vi "Wait if Occupied.vi"(9 "Desired Direction":T1, 10 "Desired Action":T2, 11 "Square":refnum<class "Square.lvclass">) -> (2 "Resulting Action":T2)   [LabVIEW 2020, in "SquareBattle.lvlib" / "Square.lvclass"]
uses:
  Square.lvclass
  Square.lvclass/Square.ctl
  Action.ctl
  SquareBattle.lvlib
  Direction.ctl
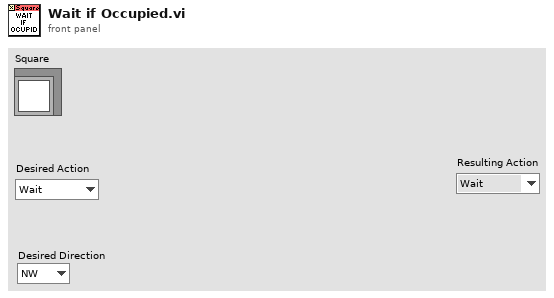
[diagram p1: front panel]
types:
  T1 = typedef "SquareBattle.lvlib/Direction.ctl" = enum16{"NW", "N", "NE", "E", "SE", "S", "SW", "W"}
  T2 = typedef "SquareBattle.lvlib/Action.ctl" = enum16{"Wait", "Move", "Attack", "Replicate"}
  T3 = typedef "SquareBattle.lvlib/Location Status.ctl" = cluster{"Empty":bool, "Friend":bool, "Enemy":bool}
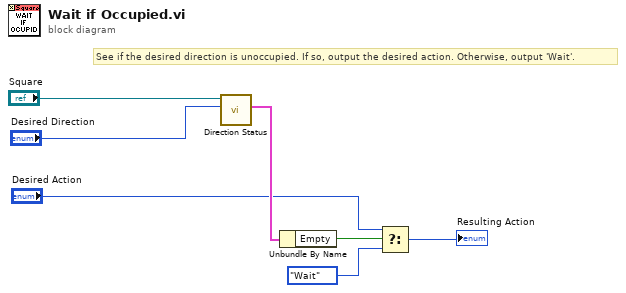
[diagram p0: block diagram]
diagram:
  # "See if the desired direction is unoccupied. If so, output the desired action. Otherwise, output 'Wait'."
  n1 = call "Direction Status.vi"("Direction"="Desired Direction", "Square"="Square") -> ("Status"=w5:T3)  [unwired: 9 in]
  n2 = Unbundle By Name(w5) -> ("Empty"=w4:bool)
  n3 = Select(t="Desired Action", s=w4, f=Action."Wait") -> (s? t:f=→"Resulting Action":T2)
